vi "Charger, Verify Storage Mode.vi"(0 "error in":errorcluster, 1 "poll delay (500 ms)":dbl[unit]=0.5, 2 "max attempts (10)":i32=10, 3 "VISA resource":refnum<visa-resource-name>="COM13", 4 "Status Refnum":T1) -> (7 "error out":errorcluster, 9 "idle":bool)   [LabVIEW 2020]
uses:
  Charger_Status Refnum.ctl
  Drivers/Charger Test Set/Charger_Input Control.ctl
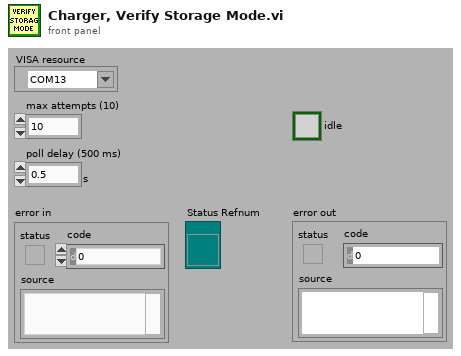
[diagram p1: front panel]
types:
  T1 = typedef "Charger_Status Refnum.ctl" = refnum<vi>
  T2 = cluster{"ERROR_OCCURRED":bool, "LINK_STAT_CHANGED":bool, "LINK_QUAL_CHANGED":bool, "400MHZ_TX_ACTIVE":bool, "400MHZ_RX_ACTIVE":bool, "245GHZ_TX_ACTIVE":bool, "DATA_STAT_CHANGED":bool, "SLEEPING":bool, "IDLE":bool, "SEARCHING_FOR_IMPLANT":bool, "STARTING_SESSION":bool, "LISTENING_FOR_EMERG":bool, "IN_SESSION":bool}
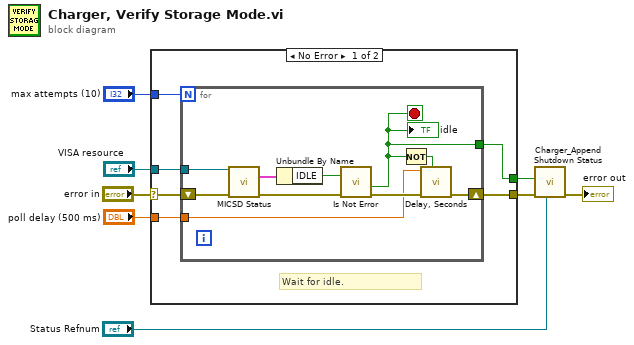
[diagram p0: block diagram]
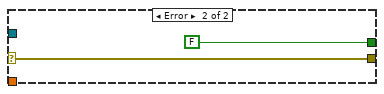
[diagram p2: hidden frame]
diagram:
  n1 = case shown="No Error" "error in" {
    selector: "error in" -> [w11 w26]
    tunnel: "VISA resource" -> [w14 _]
    tunnel: "max attempts (10)" -> [w13 _]
    tunnel: "poll delay (500 ms)" -> [w12 _]
    tunnel: [w10 w26] -> w4
    tunnel: [w9 FALSE ("ready")] -> w2
    frame No Error {
      # "Wait for idle."
      n2 = for {
        N: w13 -> [_]
        tunnel: w14 -> [w23]
        tunnel: [w17] -> w9
        tunnel: w12 -> [w16]
        shift-right: [w19] -> w10
        shift-left: w11 -> [w15]
        stop <- w17 stop-if-true
        n3 = call "MICSD Status.vi"("VISA Resource Name"=w23, "error in (no error)"=w15) -> ("Status Flags"=w24:T2, "error out"=w22:errorcluster)  [unwired: 7 in, 5 out]
        n4 = Unbundle By Name(w24) -> ("IDLE"=w20:bool)
        n5 = call "Is Not Error.vi"("enable (T)"=w20, "error in"=w22) -> ("error out"=w21:errorcluster, "ready"=w17:bool)  [unwired: 4 in, 1 out]
        "idle" <- w17
        n6 = Not(x=w17) -> (.not. x?=w18:bool)
        n7 = call "Delay, Seconds.vi"("enable (T)"=w18, "error in"=w21, "delay"=w16) -> ("error out"=w19:errorcluster)  [unwired: 4 in, 1 out]
      }
    }
    frame Error {
    }
  }
  n8 = call "Charger_Append Shutdown Status.vi"("Status Refnum"="Status Refnum", "error in"=w4, "Base Station Idle"=w2) -> ("error out"=→"error out":errorcluster)  [unwired: 6 in]
